vi "Filter(SubVI).vi"(6 "order":i32=2, 7 "filter type":T1(ring), 8 "low cutoff freq: fl":dbl=0.12500000000000006 format="%0.4f", 9 "high cutoff freq: fh":dbl=0.45000000000000007 format="%0.2f", 10 "Data":dbl[](array[numeric]), 11 "dt":dbl format="%#_13g") -> (2 "Filtered Data":dbl[](array[numeric]))   [LabVIEW 2017]
uses:
  <vilib>/Analysis/NI_AALBase.lvlib
  <vilib>/Analysis/3filter.llb/Butterworth Filter (DBL).vi
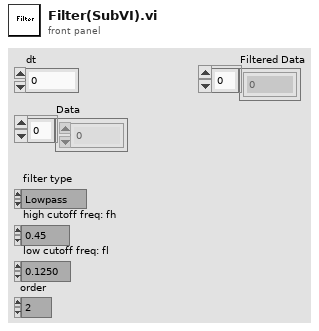
[diagram p1: front panel]
types:
  T1 = enum32{"Lowpass", "Highpass", "Bandpass", "Bandstop"}
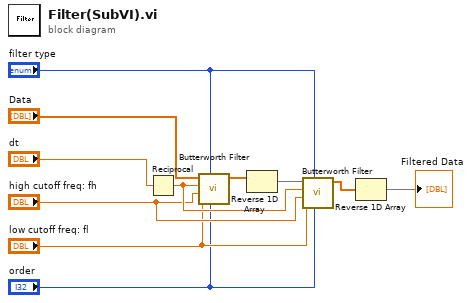
[diagram p0: block diagram]
diagram:
  n1 = Reciprocal(x="dt") -> (1/x=w8:dbl)
  n2 = call-poly <vilib>:"Butterworth Filter.vi"("order"="order", "filter type"="filter type", "low cutoff freq: fl"="low cutoff freq: fl", "high cutoff freq: fh"="high cutoff freq: fh", "sampling freq: fs"=w8, "X"="Data") -> ("Filtered X"=w11:dbl[])  [unwired: 1 in, 2 out]
  n3 = Reverse 1D Array(array=w11) -> (reversed array=w10:dbl[])
  n4 = call-poly <vilib>:"Butterworth Filter.vi"("order"="order", "filter type"="filter type", "low cutoff freq: fl"="low cutoff freq: fl", "high cutoff freq: fh"="high cutoff freq: fh", "sampling freq: fs"=w8, "X"=w10) -> ("Filtered X"=w4:dbl[])  [unwired: 1 in, 2 out]
  n5 = Reverse 1D Array(array=w4) -> (reversed array=→"Filtered Data":dbl[])
